vi "Panel.vi"(11 "WebProjectPanel in":refnum<class "WebProjectPanel.lvclass">) -> ()   [LabVIEW 2020, in "PicoG-Processor.lvlib" / "WebProjectPanel.lvclass"]
uses:
  WebProjectPanel.lvclass
  C:/Program Files (x86)/National Instruments/LabVIEW 2020/vi.lib/IlluminatedG/IG OOPanel/OOPanel/Panel/Panel.lvclass
  WebProjectPanel.lvclass/WebProjectPanel.ctl
  Get App Name.vi
  Get Last Update String.vi
  <vilib>/IlluminatedG/IG OOPanel/OOPanel/Panel/Panel.lvclass
panel:
  in  "Show Folder":bool
  in  "Deploy":bool
  out "Last Update":string
  out "Web App Name":string
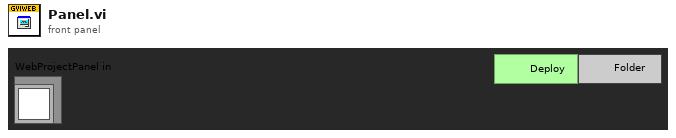
[diagram p1: front panel]
types:
  T1 = typedef "OOPanel.lvlib/Panel.lvclass/Panel Events.ctl" = cluster{"Visbility":refnum<user-event>, "Close":refnum<user-event>}
  T2 = typedef "PicoG-Processor.lvlib/WebProjectPanel.lvclass/Events.ctl" = cluster{"Updated":refnum<user-event>}
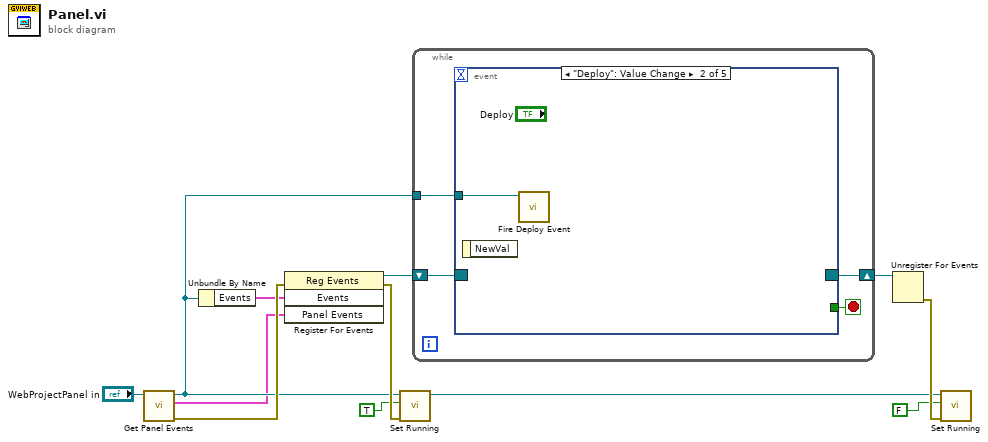
[diagram p0: block diagram]
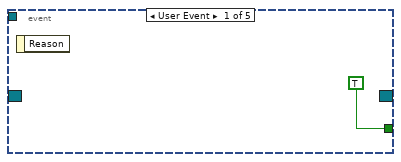
[diagram p2: hidden frame]
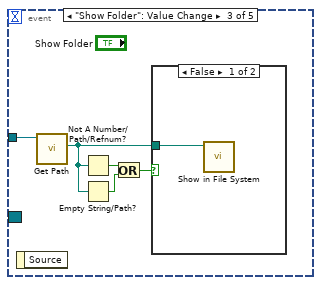
[diagram p3: hidden frame]
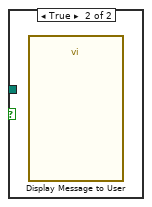
[diagram p4: hidden frame]
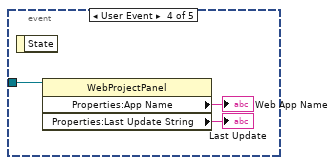
[diagram p5: hidden frame]
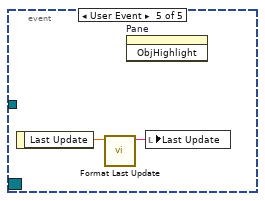
[diagram p6: hidden frame]
diagram:
  n1 = call <vilib>:"Get Panel Events.vi"("Panel in"="WebProjectPanel in") -> ("error out"=w12:errorcluster, "Panel Events"=w2:T1, "Panel out"=w4:refnum<class "WebProjectPanel.lvclass">)  [unwired: 8 in]
  n2 = Unbundle By Name(w4) -> ("Events"=w3:T2)
  n3 = register-events(error in=w12, w3, w2) -> (reference out=w10:refnum<event-registration>, error out=w8:errorcluster)  [unwired: 1 in]
  n4 = call <vilib>:"Set Running.vi"("error in (no error)"=w8, "Running"=TRUE, "Panel in"=w4) -> ("Panel out"=w1:refnum<class "WebProjectPanel.lvclass">)  [unwired: 7 in, 1 out]
  n5 = while {
    shift-right: [w15] -> w9
    shift-left: w10 -> [w16]
    tunnel: w4 -> [w13]
    stop <- w14 stop-if-true
    n6 = event shown="[1] \"Deploy\": Value Change" {
      selector: w16 -> [_ _ _ _ _]
      dyn-events: [_ _ _ _ _] -> w15
      timeout: _ -> [_ _ _ _ _]
      tunnel: [TRUE _ _ _ _] -> w14
      tunnel: w13 -> [_ w18 w23 w25 _]
      event User Event {
        n7 = event-data() -> ()  [unwired: 1 in, 1 out]
      }
      event "Deploy": Value Change {
        n8 = event-data() -> ()  [unwired: 1 in, 1 out]
        n9 = call "Fire Deploy Event.vi"("WebProjectPanel in"=w18) -> ()  [unwired: 9 in, 2 out]
      }
      event "Show Folder": Value Change {
        n10 = event-data() -> ()  [unwired: 1 in, 1 out]
        n11 = call "Get Path.vi"("WebProjectPanel in"=w23) -> ("Path"=w21:path)  [unwired: 8 in, 2 out]
        n12 = Not A Number/Path/Refnum?(number/path/refnum=w21) -> (NaN/Path/Refnum?=w22:bool)
        n13 = Empty String/Path?(string/path=w21) -> (empty?=w19:bool)
        n14 = Or(x=w22, y=w19) -> (x .or. y?=w20:bool)
        n15 = case shown="False" w20 {
          tunnel: w21 -> [w24 _]
          frame False {
            n16 = call <vilib>:"Show in File System.vi"("file or directory path"=w24) -> ()  [unwired: 10 in, 1 out]
          }
          frame True {
            n17 = call "Display Message to User"() -> ()  [unwired: 10 in, 2 out]
          }
        }
      }
      event User Event {
        n18 = event-data() -> ()  [unwired: 1 in, 1 out]
        n19 = property class="WebProjectPanel"(reference=w25) -> ("Properties:App Name"=→"Web App Name":string, "Properties:Last Update String"=→"Last Update":string)  [unwired: 1 in, 2 out]
      }
      event User Event {
        n20 = event-data() -> ("Last Update"=w29:dbl)  [unwired: 1 in]
        n21 = call "Format Last Update.vi"("Last Update"=w29) -> ("Last Update String"=w28:string)  [unwired: 10 in]
        n22 = invoke on="Pane" class="Pane" method="ObjHighlight"() -> ()  [unwired: 3 in, 3 out]
        n23 = local write "Last Update"(w28) -> ()
      }
    }
  }
  n24 = Unregister For Events(event registration refnum=w9) -> (error out=w6:errorcluster)  [unwired: 1 in]
  n25 = call <vilib>:"Set Running.vi"("error in (no error)"=w6, "Running"=FALSE, "Panel in"=w1) -> ()  [unwired: 7 in, 2 out]
